vi "Read User-Defined CSM States.vi"(8 "error in (no error)":errorcluster, 11 "CSM-Helper in":refnum<class "CSM-Helper.lvclass">) -> (0 "error out":errorcluster, 2 "Array":string[](array[string]), 3 "CSM-Helper out":refnum<class "CSM-Helper.lvclass">)   [LabVIEW 2020, in "CSM-Helper.lvclass"]
uses:
  CSM-Helper.lvclass
  CSM-Helper.lvclass/CSM-Helper.ctl
  <userlib>/_OpenG.lib/string/string.llb/Trim Whitespace (String Array)__ogtk.vi
  <userlib>/_OpenG.lib/array/array.llb/Filter 1D Array (String)__ogtk.vi
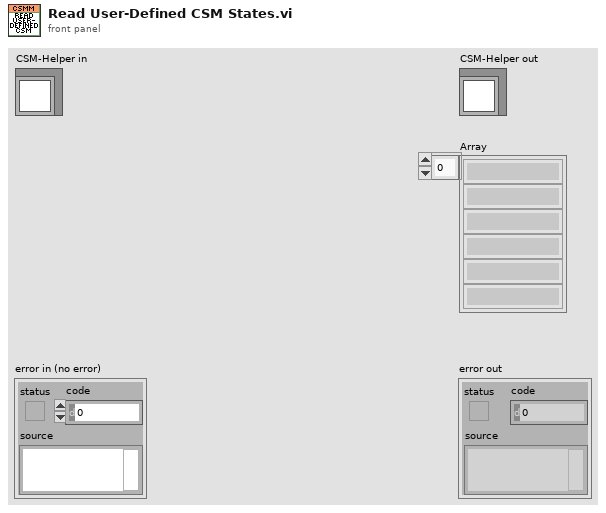
[diagram p1: front panel]
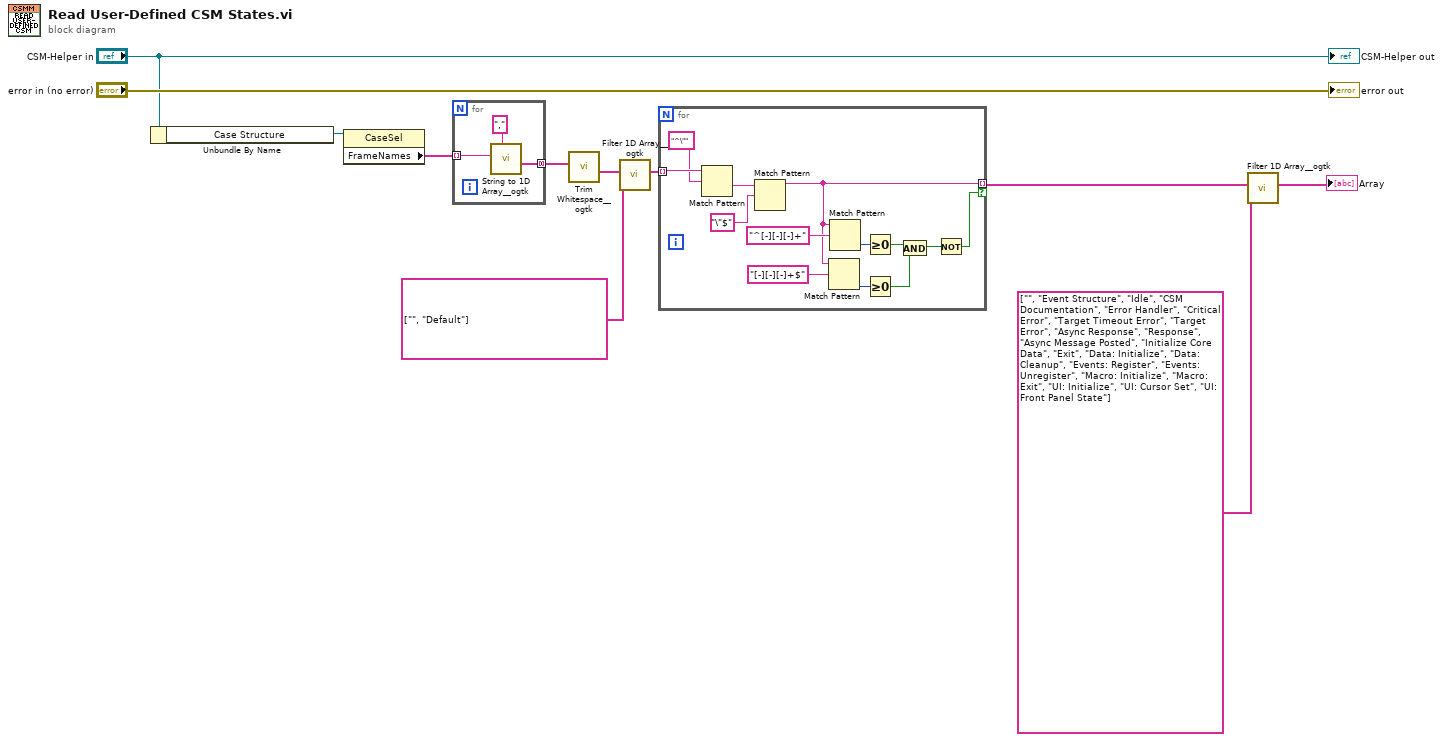
[diagram p0: block diagram]
diagram:
  n1 = Unbundle By Name("CSM-Helper in") -> ("Case Structure"=w9:refnum<vi>)
  n2 = property on="Property Node" class="CaseSel"(reference=w9) -> ("FrameNames"=w8:string[])  [unwired: 1 in, 2 out]
  n3 = for {
    tunnel: w8 -> [w14] mode=indexing
    tunnel: [w12] -> w7 mode=concatenating
    n4 = call <userlib>:"String to 1D Array__ogtk.vi"("delimiter (Tab)"=",", "string"=w14) -> ("Array of Strings"=w12:string[])  [unwired: 9 in]
  }
  n5 = call-poly <userlib>:"Trim Whitespace__ogtk.vi"("String in"=w7) -> ("String out"=w6:string[])  [unwired: 6 in]
  n6 = call-poly <userlib>:"Filter 1D Array__ogtk.vi"("items to filter"=string[] ["", "Default"], "array"=w6) -> ("filtered array"=w4:string[])  [unwired: 4 in, 1 out]
  n7 = for {
    tunnel: w4 -> [w27] mode=indexing
    tunnel: [w15] -> w2 mode=indexing if=w16
    n8 = Match Pattern(string=w27, regular expression="^\"") -> (after substring=w25:string)  [unwired: 1 in, 3 out]
    n9 = Match Pattern(string=w25, regular expression="\"$") -> (before substring=w15:string)  [unwired: 1 in, 3 out]
    n10 = Match Pattern(string=w15, regular expression="[-][-][-]+$") -> (offset past match=w20:i32)  [unwired: 1 in, 3 out]
    n11 = Match Pattern(string=w15, regular expression="^[-][-][-]+") -> (offset past match=w21:i32)  [unwired: 1 in, 3 out]
    n12 = Greater Or Equal To 0?(x=w21) -> (x >= 0?=w19:bool)
    n13 = Greater Or Equal To 0?(x=w20) -> (x >= 0?=w18:bool)
    n14 = And(x=w19, y=w18) -> (x .and. y?=w17:bool)
    n15 = Not(x=w17) -> (.not. x?=w16:bool)
  }
  n16 = call-poly <userlib>:"Filter 1D Array__ogtk.vi"("items to filter"=string[] ["", "Event Structure", "Idle", "CSM Documentation", "Error Handler", "Critical Error", "Target Timeout Error", "Target Error", "Async Response", "Response", "Async Message Posted", "Initialize Core Data", "Exit", "Data: Initialize", "Data: Cleanup", "Events: Register", "Events: Unregister", "Macro: Initialize", "Macro: Exit", "UI: Initialize", "UI: Cursor Set", "UI: Front Panel State"], "array"=w2) -> ("filtered array"=→"Array":string[])  [unwired: 4 in, 1 out]
  "error out" <- "error in (no error)"
  "CSM-Helper out" <- "CSM-Helper in"
